vi "ParseGtags.vi"(0 "tag":string, 1 "urdf in":string) -> (2 "parameters":string, 3 "not found":bool, 4 "contents":string, 5 "urdf out":string)   [LabVIEW 2010]
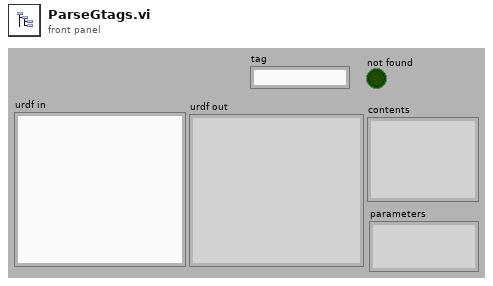
[diagram p1: front panel]
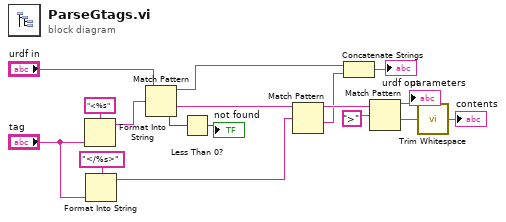
[diagram p0: block diagram]
diagram:
  n1 = Format Into String(format string="<%s" ("regular expression"), "tag") -> (resulting string=w4:string)  [unwired: 2 in, 1 out]
  n2 = Format Into String(format string="</%s>" ("regular expression"), "tag") -> (resulting string=w13:string)  [unwired: 2 in, 1 out]
  n3 = Match Pattern(string="urdf in", regular expression=w4) -> (before substring=w7:string, after substring=w9:string, offset past match=w2:i32)  [unwired: 1 in, 1 out]
  n4 = Less Than 0?(x=w2) -> (x < 0?=→"not found":bool)
  n5 = Match Pattern(string=w9, regular expression=w13) -> (before substring=w14:string, after substring=w6:string)  [unwired: 1 in, 2 out]
  n6 = Concatenate Strings(w7, w6) -> (→"urdf out":string)
  n7 = Match Pattern(string=w14, regular expression=">") -> (before substring=→"parameters":string, after substring=w16:string)  [unwired: 1 in, 2 out]
  n8 = call <vilib>:"Trim Whitespace.vi"("string"=w16) -> ("trimmed string"=→"contents":string)  [unwired: 1 in]
